vi "Read Device Identification.vi"(8 "error in (no error)":errorcluster, 9 "read device ID code":T1, 10 "object ID":u8, 11 "Modbus slave in":refnum<class "Modbus Master CR API.lvclass">) -> (0 "error out":errorcluster, 2 "objects":cluster{"object ID":u8, "value":string}[](array[cluster]) {"object ID" format="%x"}, 3 "Modbus slave out":refnum<class "Modbus Master CR API.lvclass">)   [LabVIEW 2021, in "Modbus Master CR API.lvclass"]
doc: "Returns the device identification of a Modbus slave. Device identification consists of data elements called objects. Each object has an identification number and stores Modbus slave information."
uses:
  Modbus Master CR API.lvclass
  Modbus Master CR API.lvclass/Modbus Master CR API.ctl
  Data Model/Device Data Model.lvclass
  Master Function Definition/Read Device ID code.ctl
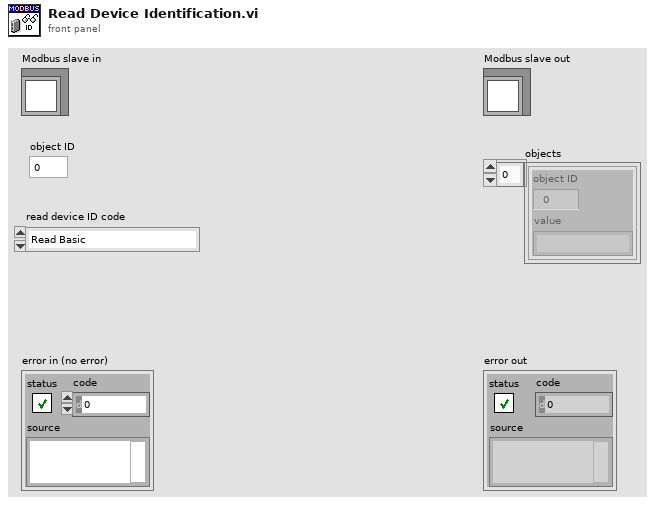
[diagram p1: front panel]
types:
  T1 = typedef "Device Data Model.lvclass/Read Device ID code.ctl" = enum8{"Read Basic", "Read Regular", "Read Extended", "Read Specific"}
  T2 = typedef "Device Data Model.lvclass/Identification Parameters.ctl" = cluster{"Object ID":u8, "Value":string}
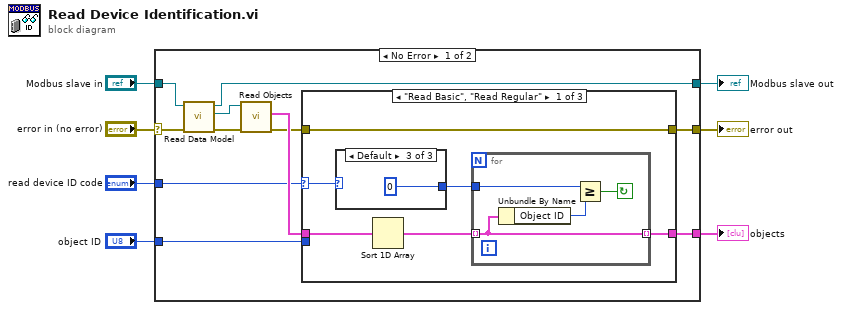
[diagram p0: block diagram]
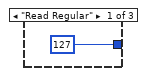
[diagram p2: hidden frame]
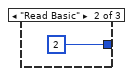
[diagram p3: hidden frame]
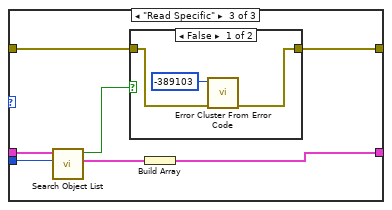
[diagram p5: hidden frame]
diagram:
  n1 = case shown="No Error" "error in (no error)" {
    selector: "error in (no error)" -> [w12 w45]
    tunnel: [w9 w46] -> w7
    tunnel: "Modbus slave in" -> [w8 w46]
    tunnel: "read device ID code" -> [w17 _]
    tunnel: "object ID" -> [w16 _]
    tunnel: [w15 _] -> w4
    tunnel: [w14 w45] -> w3
    frame No Error {
      n2 = call "Read Data Model.vi"("error in (no error)"=w12, "Modbus slave in"=w8) -> ("error out"=w11:errorcluster, "device data model"=w10:refnum<class "Device Data Model.lvclass">, "Modbus slave out"=w9:refnum<class "Modbus Master CR API.lvclass">)  [unwired: 7 in]
      n3 = call-dynamic "Read Objects.vi"("error in"=w11, "device data model in"=w10) -> ("error out"=w13:errorcluster, "Objects"=w18:T2[])  [unwired: 7 in, 1 out]
      n4 = case shown="\"Read Basic\", \"Read Regular\"" w17 {
        selector: w17 -> [w21 _ _]
        tunnel: w18 -> [w22 w32 w40]
        tunnel: w13 -> [w24 w33 w35]
        tunnel: w16 -> [_ _ w39]
        tunnel: [w23 w32 w36] -> w15
        tunnel: [w24 w33 w34] -> w14
        frame "Read Basic", "Read Regular" {
          n5 = case shown="Default" w21 {
            tunnel: [u8 127 ("y") u8 2 ("y") u8 0 ("y")] -> w20
            frame "Read Regular" {
            }
            frame "Read Basic" {
            }
            frame Default {
            }
          }
          n6 = Sort 1D Array(array=w22) -> (sorted array=w19:T2[])
          n7 = for {
            tunnel: w19 -> [w31] mode=indexing
            tunnel: [w31] -> w23 mode=indexing
            tunnel: w20 -> [w29]
            stop <- w30 continue-if-true
            n8 = Unbundle By Name(w31) -> ("Object ID"=w28:u8)
            n9 = Greater Or Equal?(x=w29, y=w28) -> (x >= y?=w30:bool)
          }
        }
        frame "Read Extended" {
        }
        frame "Read Specific" {
          n10 = call "Search Object List.vi"("Object ID"=w39, "Objects"=w40) -> ("Object"=w37:T2, "Found?"=w38:bool)  [unwired: 7 in, 1 out]
          n11 = case shown="False" w38 {
            tunnel: w35 -> [w42 w44]
            tunnel: [w43 w44] -> w34
            frame False {
              n12 = call <vilib>:"Error Cluster From Error Code.vi"("error in (no error)"=w42, "error code (0)"=-389103) -> ("error out"=w43:errorcluster)  [unwired: 7 in]
            }
            frame True {
            }
          }
          n13 = Build Array(w37) -> (w36:T2[])
        }
      }
    }
    frame Error {
    }
  }
  "error out" <- w3
  "Modbus slave out" <- w7
  "objects" <- w4
